vi "Get Event Timing Captures - Multi FPGA.vi"(0 "Item Ref in":T2 format="%.0x", 1 "Window":string, 5 "Timing measurement":string, 7 "return all captures (T)":bool=TRUE, 11 "error in (no error)":errorcluster) -> (2 "window":T1, 3 "not present indexes":i32[](array[numeric]), 4 "Item Ref out":T2 format="%.0x", 6 "captures":T3[](array[typedef]), 8 "window found":bool, 10 "Window reference angle":dbl, 12 "Capture item refs":T2[](array[typedef]) format="%.0x", 14 "degrees of one u16":dbl, 15 "error out":errorcluster)   [LabVIEW 2015, in "Engine Simulation Toolkit System Explorer.lvlib"]
uses:
  Engine Simulation Toolkit System Explorer.lvlib
  Event Timing Capture.ctl
  Event Reference Angle Selection.ctl
  <vilib>/NI Veristand/Custom Device API/Custom Device Item Ref.ctl
  Event Timing Window.ctl
  <vilib>/NI Veristand/Custom Device Tools/Custom Device Utility Library/Search Direction.ctl
  Shared/Properties.vi
  Shared/Constants and GUIDs.vi
  <vilib>/NI Veristand/Custom Device Tools/Custom Device Utility Library/NI VeriStand - Search for Item by GUID.vi
  <vilib>/NI Veristand/Custom Device Tools/Custom Device Utility Library/NI VeriStand - Search for All Items by GUID.vi
  <vilib>/NI Veristand/Custom Device API/Get Item Property (String).vi
  <vilib>/NI Veristand/Custom Device API/Get Item Property (Double).vi
  <vilib>/NI Veristand/Custom Device API/Get Item Property (U16).vi
  Shared/Engine Simulation Toolkit Shared.lvlib
  <vilib>/NI Veristand/Custom Device API/Custom Device API.lvlib
  <vilib>/NI Veristand/Custom Device Tools/Custom Device Utility Library/Custom Device Utility Library.lvlib
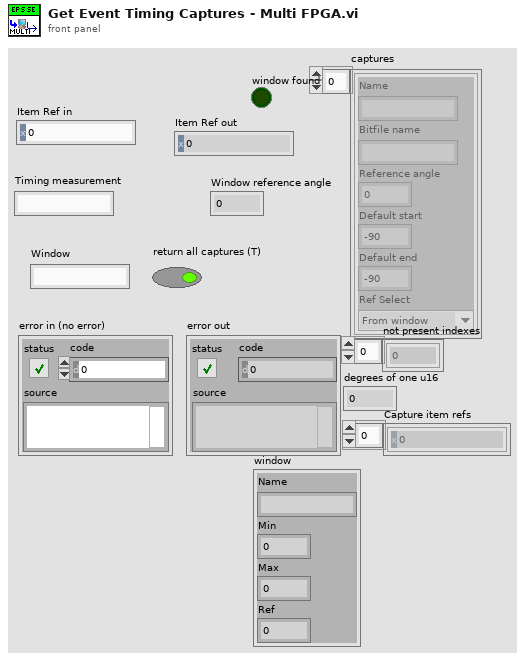
[diagram p1: front panel]
types:
  T1 = typedef "Engine Simulation Toolkit System Explorer.lvlib/Event Timing Window.ctl" = cluster{"Name":string, "Min":dbl, "Max":dbl, "Ref":dbl}
  T2 = typedef "Custom Device API.lvlib/Custom Device Item Ref.ctl" = u64
  T3 = typedef "Engine Simulation Toolkit System Explorer.lvlib/Event Timing Capture.ctl" = cluster{"Name":string, "Bitfile name":string, "Reference angle":dbl, "Default start":dbl, "Default end":dbl, "Ref Select":T4}
  T4 = typedef "Engine Simulation Toolkit System Explorer.lvlib/Event Reference Angle Selection.ctl" = enum16{"From window", "Custom"}
  T5 = typedef "Custom Device Utility Library.lvlib/Search Direction.ctl" = enum16{"Down", "Up"}
  T6 = typedef "Custom Device API.lvlib/Custom Device Item Info.ctl" = cluster{"Name":string, "Is Channel":bool, "GUID":string, "Is Waveform":bool}
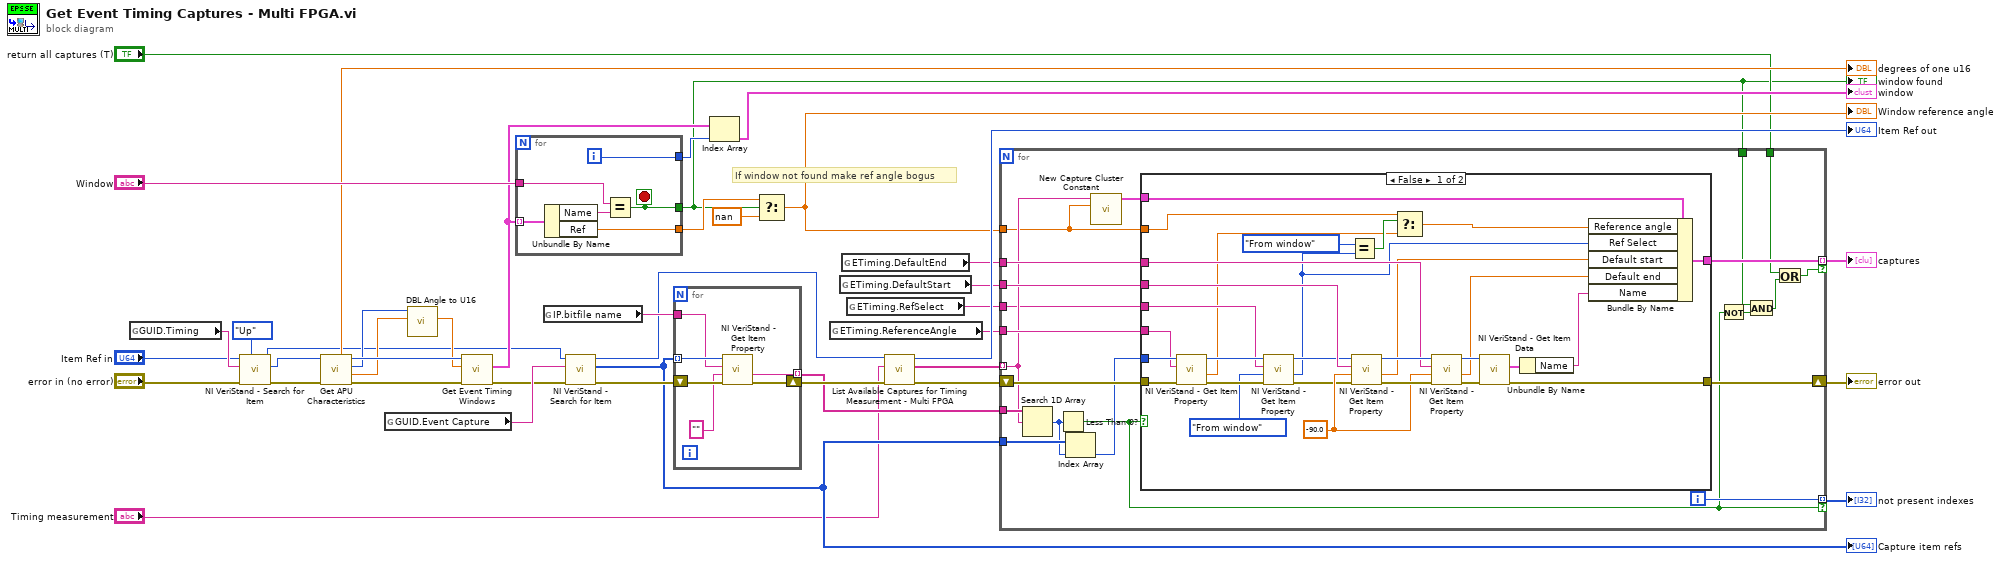
[diagram p0: block diagram]
diagram:
  # "If window not found make ref angle bogus"
  n1 = global read "Constants and GUIDs.vi" "GUID.Timing"() -> (w5:string)
  n2 = call-poly <vilib>:"NI VeriStand - Search for Item.vi"("Direction (Down)"=Search_Direction."Up", "error in"="error in (no error)", "Item GUID"=w5, "Section Ref in"="Item Ref in") -> ("error out"=w6:errorcluster, "Item Ref"=w3:T2, "Section Ref out"=w1:T2)  [unwired: 4 in, 1 out]
  n3 = call "Get APU Characteristics.vi"("error in (no error)"=w6, "Item Ref in"=w3) -> ("error out"=w24:errorcluster, "angle to u16 scale factor"=w20:dbl, "total angle span (degrees)"=w21:u16, "Item Ref out"=w23:T2, "degrees of one u16"=→"degrees of one u16":dbl)  [unwired: 3 in, 2 out]
  n4 = global read "Constants and GUIDs.vi" "GUID.Event Capture"() -> (w25:string)
  n5 = call "DBL Angle to U16.vi"("angle to u16 scale factor"=w20, "Desired angle (degrees)"=w21) -> ("Actual angle (degrees)"=w22:dbl)  [unwired: 8 in, 1 out]
  n6 = call "Get Event Timing Windows.vi"("error in (no error)"=w24, "Max engine angle"=w22, "Item Ref in"=w23) -> ("error out"=w19:errorcluster, "Windows"=w12:T1[])  [unwired: 6 in, 1 out]
  n7 = for {
    tunnel: w12 -> [w47] mode=indexing
    tunnel: "Window" -> [w45]
    tunnel: [w44] -> w16
    tunnel: [w43] -> w8
    tunnel: [w42] -> w11
    i -> [w42]
    stop <- w43 stop-if-true
    n8 = Unbundle By Name(w47) -> ("Name"=w46:string, "Ref"=w44:dbl)
    n9 = Equal?(x=w45, y=w46) -> (x = y?=w43:bool)
  }
  "window found" <- w8
  n10 = global read "Properties.vi" "IP.bitfile name"() -> (w32:string)
  n11 = call-poly <vilib>:"NI VeriStand - Search for Item.vi"("error in"=w19, "Item GUID"=w25, "Section Ref in"=w1) -> ("error out"=w33:errorcluster, "Item Refs"=w28:T2[], "Section Ref out"=w31:T2)  [unwired: 5 in, 1 out]
  "Capture item refs" <- w28
  n12 = for {
    shift-right: [w50] -> w30
    shift-left: w33 -> [w53]
    tunnel: w28 -> [w52] mode=indexing
    tunnel: w32 -> [w51]
    tunnel: [w48] -> w29 mode=indexing
    n13 = call-poly <vilib>:"NI VeriStand - Get Item Property.vi"("error in (no error)"=w53, "Default Value"="", "Property Name"=w51, "Item Ref in"=w52) -> ("error out"=w50:errorcluster, "Value"=w48:string)  [unwired: 4 in, 2 out]
  }
  n14 = Index Array(array=w12, index=w11) -> (element=→"window":T1)
  n15 = Select(t=w16, s=w8, f=nan) -> (s? t:f=w14:dbl)
  "Window reference angle" <- w14
  n16 = global read "Properties.vi" "ETiming.ReferenceAngle"() -> (w36:string)
  n17 = global read "Properties.vi" "ETiming.DefaultStart"() -> (w35:string)
  n18 = global read "Properties.vi" "ETiming.DefaultEnd"() -> (w27:string)
  n19 = global read "Properties.vi" "ETiming.RefSelect"() -> (w17:string)
  n20 = call "List Available Captures for Timing Measurement - Multi FPGA.vi"("error in (no error)"=w30, "Timing measurement"="Timing measurement", "Item Ref in"=w31) -> ("error out"=w40:errorcluster, "captures available"=w39:string[], "Item Ref out"=→"Item Ref out":T2)  [unwired: 6 in]
  n21 = for {
    tunnel: [w62] -> w41 mode=indexing if=w59
    shift-right: [w72] -> w37
    shift-left: w40 -> [w70]
    tunnel: w39 -> [w63] mode=indexing
    tunnel: w36 -> [w74]
    tunnel: w35 -> [w73]
    tunnel: [w71] -> w34 mode=indexing if=w56
    tunnel: w29 -> [w69]
    tunnel: w28 -> [w68]
    tunnel: w27 -> [w65]
    tunnel: w17 -> [w61]
    tunnel: w14 -> [w60]
    tunnel: "return all captures (T)" -> [w58]
    tunnel: w8 -> [w54]
    i -> [w71]
    n22 = Search 1D Array(1D array=w69, element=w63) -> (index of element=w67:i32)  [unwired: 1 in]
    n23 = Less Than 0?(x=w67) -> (x < 0?=w56:bool)
    n24 = Index Array(array=w68, index=w67) -> (element=w66:T2)
    n25 = call "New Capture Cluster Constant.vi"("Window ref angle"=w60, "Bitfile name"=w63) -> ("Capture"=w64:T3)  [unwired: 9 in]
    n26 = case shown="False" w56 {
      tunnel: w70 -> [w103 w105]
      tunnel: w66 -> [w102 _]
      tunnel: w74 -> [w101 _]
      tunnel: w73 -> [w99 _]
      tunnel: [w97 w105] -> w72
      tunnel: w65 -> [w92 _]
      tunnel: w64 -> [w91 w104]
      tunnel: [w87 w104] -> w62
      tunnel: w61 -> [w82 _]
      tunnel: w60 -> [w77 _]
      frame False {
        w86 = -90.0
        n27 = call-poly <vilib>:"NI VeriStand - Get Item Property.vi"("error in (no error)"=w103, "Property Name"=w101, "Item Ref in"=w102) -> ("error out"=w100:errorcluster, "Value"=w78:dbl, "Item Ref out"=w84:T2)  [unwired: 5 in, 1 out]
        n28 = call-poly <vilib>:"NI VeriStand - Get Item Property.vi"("error in (no error)"=w100, "Default Value"=Event_Reference_Angle_Selection."From window" ("Reference angle"), "Property Name"=w82, "Item Ref in"=w84) -> ("error out"=w85:errorcluster, "Value"=w75:u16, "Item Ref out"=w83:T2)  [unwired: 4 in, 1 out]
        n29 = Equal?(x=Event_Reference_Angle_Selection."From window" ("Reference angle"), y=w75) -> (x = y?=w79:bool)
        n30 = call-poly <vilib>:"NI VeriStand - Get Item Property.vi"("error in (no error)"=w85, "Default Value"=w86, "Property Name"=w99, "Item Ref in"=w83) -> ("error out"=w98:errorcluster, "Value"=w90:dbl, "Item Ref out"=w94:T2)  [unwired: 4 in, 1 out]
        n31 = Select(t=w77, s=w79, f=w78) -> (s? t:f=w76:dbl)
        n32 = call-poly <vilib>:"NI VeriStand - Get Item Property.vi"("error in (no error)"=w98, "Default Value"=w86, "Property Name"=w92, "Item Ref in"=w94) -> ("error out"=w95:errorcluster, "Value"=w89:dbl, "Item Ref out"=w93:T2)  [unwired: 4 in, 1 out]
        n33 = call <vilib>:"NI VeriStand - Get Item Data.vi"("error in (no error)"=w95, "Item Ref in"=w93) -> ("error out"=w97:errorcluster, "Item Info"=w96:T6)  [unwired: 6 in, 2 out]
        n34 = Unbundle By Name(w96) -> ("Name"=w88:string)
        n35 = Bundle By Name(cluster=w91, "Reference angle"=w76, "Ref Select"=w75, "Default start"=w90, "Default end"=w89, "Name"=w88) -> (w87:T3)
      }
      frame True {
      }
    }
    n36 = Not(x=w56) -> (.not. x?=w57:bool)
    n37 = And(x=w54, y=w57) -> (x .and. y?=w55:bool)
    n38 = Or(x=w58, y=w55) -> (x .or. y?=w59:bool)
  }
  "error out" <- w37
  "captures" <- w41
  "not present indexes" <- w34
